vi "unix time 1s.vi"() -> (0 "time stamp":timestamp, 1 "unix time (ms)":u64)   [LabVIEW 2019, in "Timers.lvlib"]
uses:
  Timers.lvlib
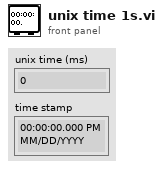
[diagram p1: front panel]
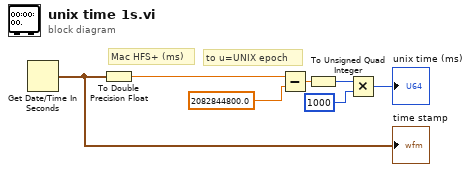
[diagram p0: block diagram]
diagram:
  # "to u=UNIX epoch"
  # "Mac HFS+ (ms)"
  n1 = Get Date/Time In Seconds() -> (seconds since 1Jan1904=w6:timestamp)
  "time stamp" <- w6
  n2 = To Double Precision Float(number=w6) -> (double precision float=w1:dbl)
  n3 = Subtract(x=w1, y=2082844800.0) -> (x-y=w5:dbl)
  n4 = To Unsigned Quad Integer(1:w5) -> (0:w3:u64)
  n5 = Multiply(x=w3, y=u64 1000) -> (x*y=→"unix time (ms)":u64)
